vi "GetAttributes.vi"(8 "error in (no error)":errorcluster, 11 "BrowerComponent in":refnum<class "BrowerComponent.lvclass">) -> (0 "error out":errorcluster, 2 "Attributes":variant, 3 "BrowerComponent out":refnum<class "BrowerComponent.lvclass">)   [LabVIEW 2015, in "BrowerComponent.lvclass"]
uses:
  BrowerComponent.lvclass
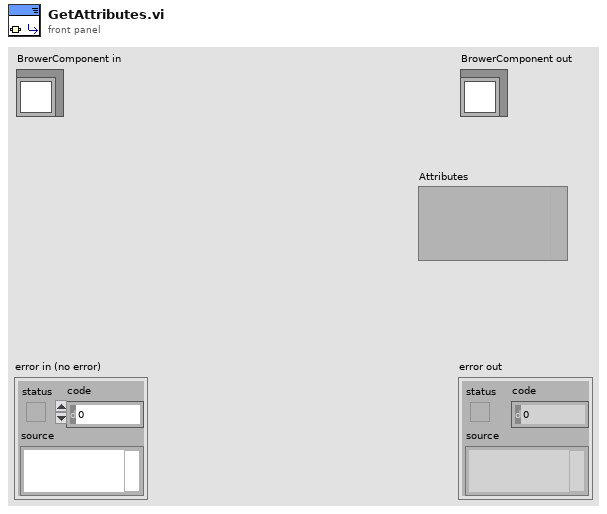
[diagram p1: front panel]
types:
  T1 = typedef "BrowerComponent.lvclass/ObjectAttributes.ctl" = cluster{"ComponentID":string, "SymbolIndex":i32, "ComponentName":string, "PartsOfComponent_dict":variant}
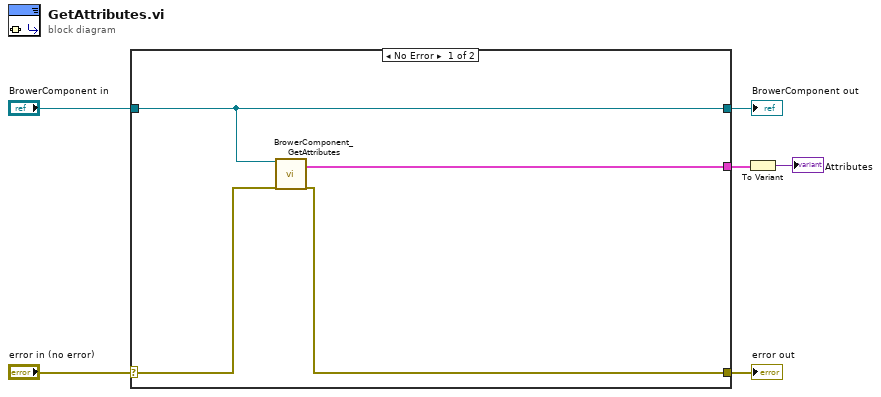
[diagram p0: block diagram]
diagram:
  n1 = case shown="No Error" "error in (no error)" {
    selector: "error in (no error)" -> [w9 w12]
    tunnel: [w7 w12] -> w5
    tunnel: [w10 w11] -> w3
    tunnel: "BrowerComponent in" -> [w10 w11]
    tunnel: [w8 _] -> w2
    frame No Error {
      n2 = call "BrowerComponent_GetAttributes.vi"("reference in"=w10, "error in (no error)"=w9) -> ("Data"=w8:T1, "error out"=w7:errorcluster)  [unwired: 14 in, 2 out]
    }
    frame Error {
    }
  }
  "error out" <- w5
  "BrowerComponent out" <- w3
  n3 = To Variant(anything=w2) -> (Variant=→"Attributes":variant)
